vi "IVC_OC200_read.vi"(6 "Channel":i32, 8 "error in (no error)":errorcluster, 11 "VISA Refnum in":refnum<visa-resource-name>="COM7") -> (0 "error out":errorcluster, 1 "read buffer":string, 2 "Status":bool, 3 "VISA Refnum out":refnum<visa-resource-name>, 4 "return count":u32, 7 "IVC (Torr)":dbl)   [LabVIEW 2019]
panel:
  out "IVC  (HPa)":dbl
  out "x-y":dbl
  out "exponent":string
  out "Mantissa":string
  out "VISA resource name out":refnum<visa-resource-name>
  out "substring":string
  out "x-y*floor(x/y)":u64
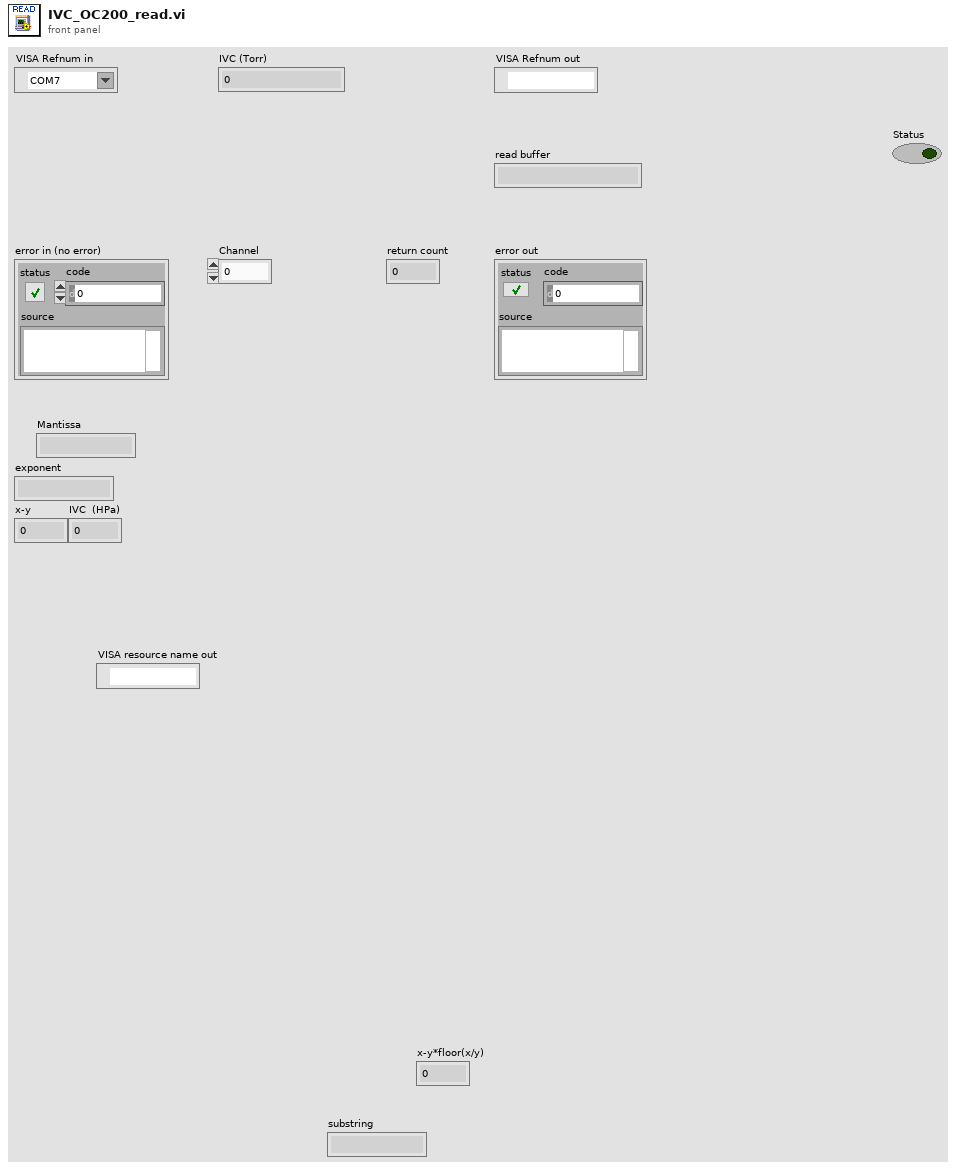
[diagram p1: front panel]
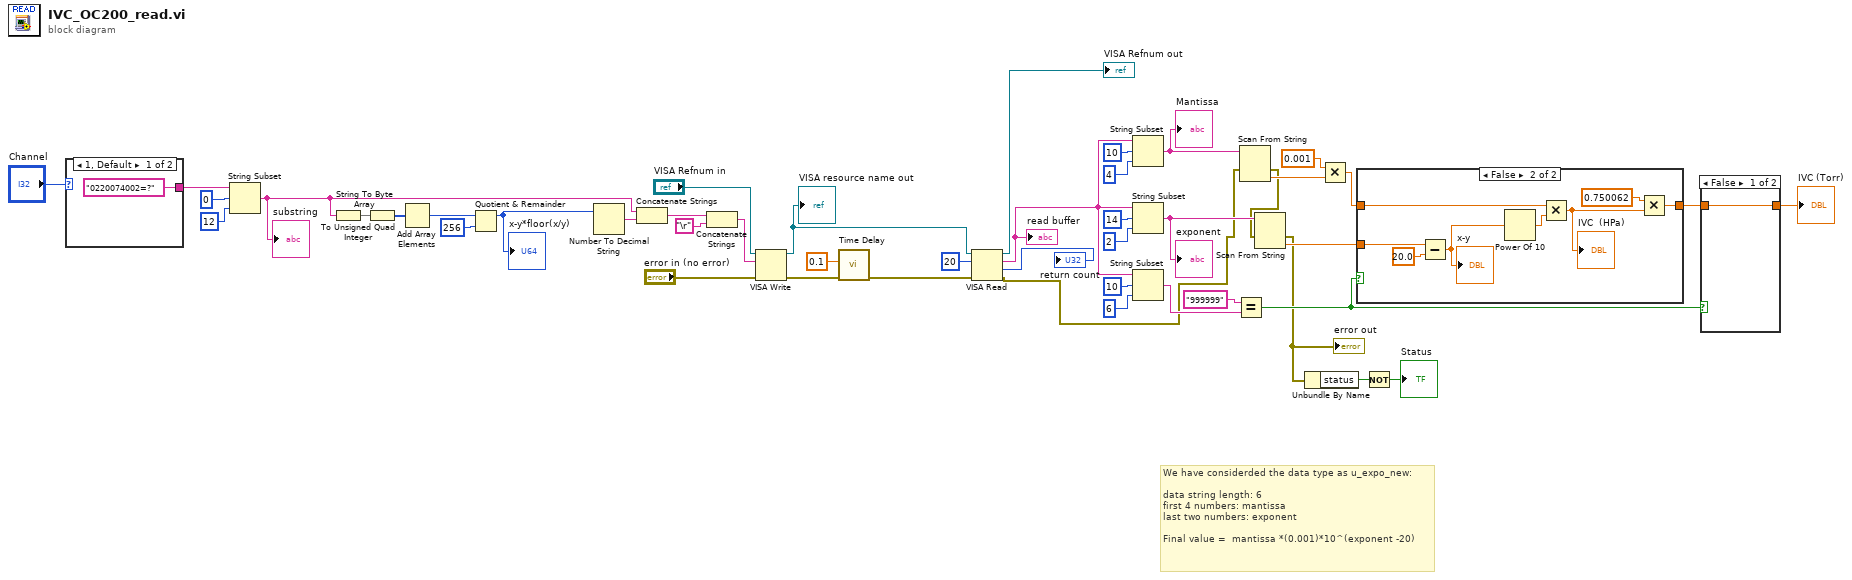
[diagram p0: block diagram]
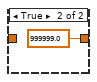
[diagram p3: hidden frame]
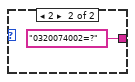
[diagram p4: hidden frame]
diagram:
  # "We have considerded the data type as u_expo_new:\n\ndata string length: 6\nfirst 4 numbers: mantissa\nlast two numbers: exponent\n\nFinal value =  mantissa *(0.001)*10^(exponent -20)"
  n1 = case shown="1, Default" "Channel" {
    tunnel: ["0220074002=?" "0320074002=?"] -> w23
    frame 1, Default {
    }
    frame 2 {
    }
  }
  n2 = String Subset(string=w23, offset (0)=0, length (rest)=12 ("length (rest)")) -> (substring=w27:string)
  "substring" <- w27
  n3 = String To Byte Array(string=w27) -> (unsigned byte array=w30:u8[])
  n4 = To Unsigned Quad Integer(1:w30) -> (0:w31:u64[])
  n5 = Add Array Elements(numeric array=w31) -> (sum=w29:u64)
  n6 = Quotient & Remainder(x=w29, y=u64 256) -> (x-y*floor(x/y)=w25:u64)  [unwired: 1 out]
  "x-y*floor(x/y)" <- w25
  n7 = Number To Decimal String(number=w25) -> (decimal integer string=w26:string)  [unwired: 1 in]
  n8 = Concatenate Strings(w27, w26) -> (w24:string)
  n9 = Concatenate Strings(w24, "\r") -> (w43:string)
  n10 = VISA Write(VISA resource name="VISA Refnum in", write buffer=w43, error in (no error)="error in (no error)") -> (VISA resource name out=w40:refnum<visa-resource-name>, error out=w42:errorcluster)  [unwired: 1 out]
  "VISA resource name out" <- w40
  n11 = call "Time Delay"("error in (no error)"=w42, "Delay Time (s)"=0.1) -> ("error out"=w37:errorcluster)  [unwired: 9 in]
  n12 = VISA Read(VISA resource name=w40, byte count=u32 20, error in (no error)=w37) -> (VISA resource name out=→"VISA Refnum out":refnum<visa-resource-name>, read buffer=w13:string, return count=→"return count":u32, error out=w3:errorcluster)
  "read buffer" <- w13
  n13 = String Subset(string=w13, offset (0)=10, length (rest)=4 ("length (rest)")) -> (substring=w21:string)
  "Mantissa" <- w21
  n14 = String Subset(string=w13, offset (0)=14, length (rest)=2 ("length (rest)")) -> (substring=w17:string)
  "exponent" <- w17
  n15 = String Subset(string=w13, offset (0)=10, length (rest)=6 ("length (rest)")) -> (substring=w11:string)
  n16 = Equal?(x="999999", y=w11) -> (x = y?=w6:bool)
  n17 = Scan From String(input string=w21, error in=w3) -> (error out=w4:errorcluster, output 1=w19:dbl)  [unwired: 3 in, 2 out]
  n18 = Scan From String(input string=w17, error in=w4) -> (error out=w2:errorcluster, output 1=w7:dbl)  [unwired: 3 in, 2 out]
  "error out" <- w2
  n19 = Unbundle By Name(w2) -> ("status"=w5:bool)
  n20 = Multiply(x=0.001, y=w19) -> (x*y=w16:dbl)
  n21 = case shown="False" w6 {
    tunnel: w16 -> [w49 w55]
    tunnel: [w49 w52] -> w8
    tunnel: w7 -> [_ w50]
    frame True {
    }
    frame False {
      n22 = Subtract(x=w50, y=20.0) -> (x-y=w57:dbl)
      "x-y" <- w57
      n23 = Power Of 10(x=w57) -> (10^x=w56:dbl)
      n24 = Multiply(x=w55, y=w56) -> (x*y=w53:dbl)
      "IVC  (HPa)" <- w53
      n25 = Multiply(x=0.750062 ("y"), y=w53) -> (x*y=w52:dbl)
    }
  }
  n26 = Not(x=w5) -> (.not. x?=→"Status":bool)
  n27 = case shown="False" w6 {
    tunnel: w8 -> [w58 _]
    tunnel: [w58 999999.0] -> w12
    frame False {
    }
    frame True {
    }
  }
  "IVC (Torr)" <- w12
